vi "Add Integers.vi"(10 "B":i64, 11 "A":i64) -> (3 "A+B":i64)   [LabVIEW 2024]
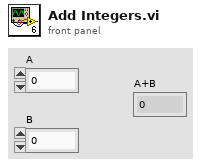
[diagram p1: front panel]
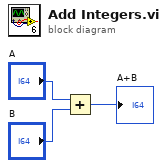
[diagram p0: block diagram]
diagram:
  n1 = Add(x="A", y="B") -> (x+y=→"A+B":i64)
